vi "Read Database.vi"(8 "error in (no error)":errorcluster, 11 "Message in":refnum<class "String Database.lvclass">=refnum) -> (0 "error out":errorcluster, 2 "Database":variant, 3 "Message out":refnum<class "String Database.lvclass">)   [LabVIEW 2018, in "String Database.lvlib" / "String Database.lvclass"]
uses:
  String Database.lvclass
  String Database.lvclass/String Database.ctl
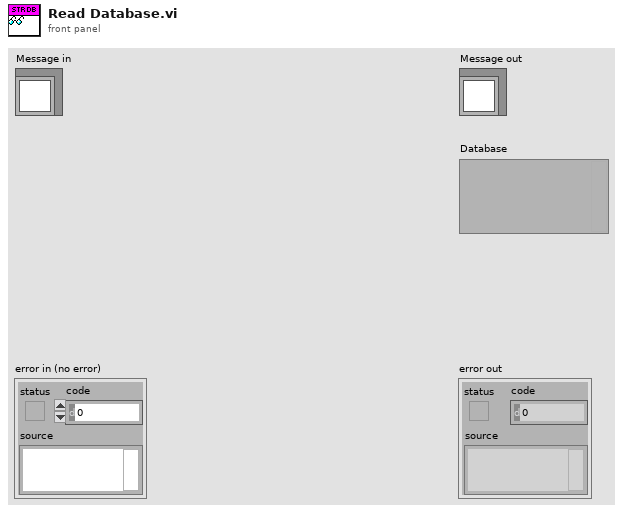
[diagram p1: front panel]
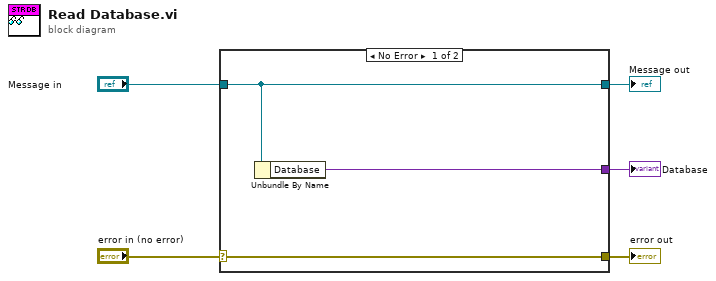
[diagram p0: block diagram]
diagram:
  n1 = case shown="No Error" "error in (no error)" {
    selector: "error in (no error)" -> [w8 w9]
    tunnel: [w8 w9] -> w4
    tunnel: [w7 w10] -> w2
    tunnel: "Message in" -> [w7 w10]
    tunnel: [w6 _] -> w1
    frame No Error {
      n2 = Unbundle By Name(w7) -> ("Database"=w6:variant)
    }
    frame Error {
    }
  }
  "error out" <- w4
  "Message out" <- w2
  "Database" <- w1
